vi "Test - Execute Step.vi"(8 "error in (no error)":errorcluster, 11 "Cluster":T1={"Preslip Sequence"=[], "Step No"=0, "Step Value"={"Sr.no"=0, "Log?"=FALSE, "Step"="", "Type"="", "Channel"="", "Value"=0.0, "Para1"=0.0, "Para2"=0.0, "Limit1"=0.0, "Limit2"=0.0, "Comparision Mode"="", "Timeout"=0.0}, "Slip Parameter"=[], "Slip Timer"=0.0, "Postslip Sequence"=[], "Postslip ?"=FALSE, "Step Result"={"Step Name"="", "Value"=0.0, "Success ?"=TRUE, "Stop Seq ?"=TRUE, "Abort"=TRUE, "Sr.No"=0}}) -> (0 "error out":errorcluster, 3 "output cluster":T1={"Preslip Sequence"=[], "Step No"=0, "Step Value"={"Sr.no"=0, "Log?"=FALSE, "Step"="", "Type"="", "Channel"="", "Value"=0.0, "Para1"=0.0, "Para2"=0.0, "Limit1"=0.0, "Limit2"=0.0, "Comparision Mode"="", "Timeout"=0.0}, "Slip Parameter"=[], "Slip Timer"=0.0, "Postslip Sequence"=[], "Postslip ?"=FALSE, "Step Result"={"Step Name"="", "Value"=0.0, "Success ?"=TRUE, "Stop Seq ?"=TRUE, "Abort"=TRUE, "Sr.No"=0}})   [LabVIEW 2017]
uses:
  Test - Message cluster.ctl
  Test - Step config.ctl
  Test - Step Result.ctl
  Controls/RT- Get Set.ctl
  Controls/RT- Queue States.ctl
  DAQ/DAQ -Driver Control.ctl
  SubVIs/SubVI - Global.vi
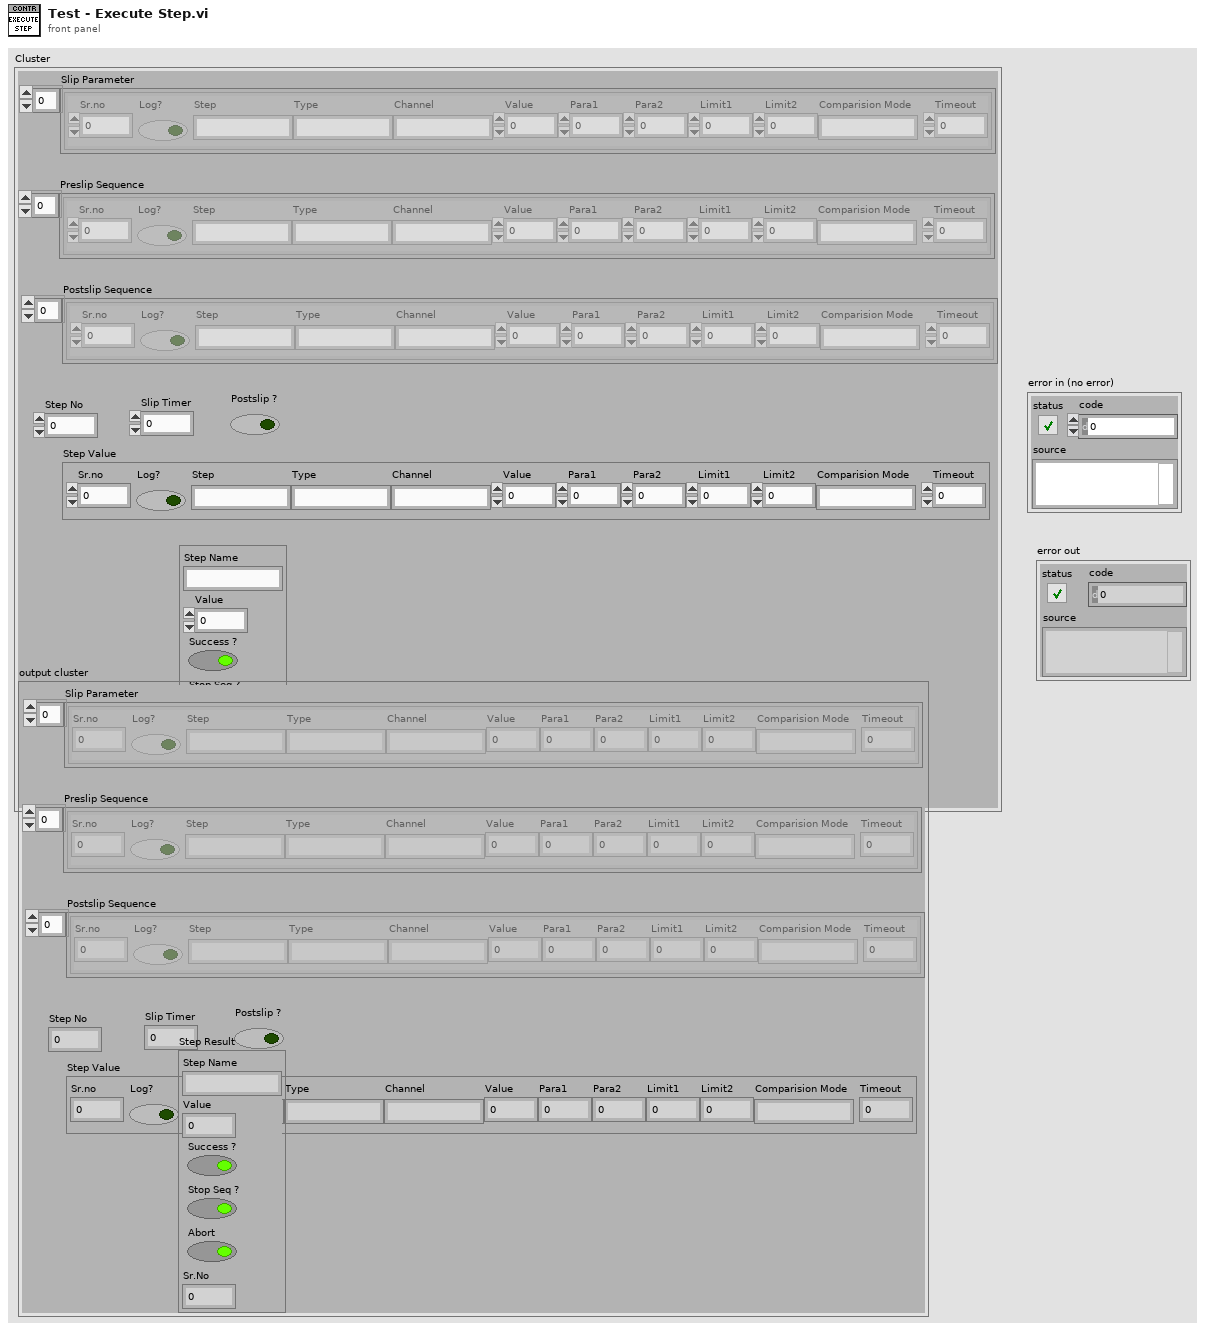
[diagram p1: front panel]
types:
  T1 = typedef "Test - Message cluster.ctl" = cluster{"Preslip Sequence":T2[], "Step No":i32, "Step Value":T2, "Slip Parameter":T2[], "Slip Timer":dbl, "Postslip Sequence":T2[], "Postslip ?":bool, "Step Result":T3}
  T2 = typedef "Test - Step config.ctl" = cluster{"Sr.no":i32, "Log?":bool, "Step":string, "Type":string, "Channel":string, "Value":dbl, "Para1":dbl, "Para2":dbl, "Limit1":dbl, "Limit2":dbl, "Comparision Mode":string, "Timeout":dbl}
  T3 = typedef "Test - Step Result.ctl" = cluster{"Step Name":string, "Value":dbl, "Success ?":bool, "Stop Seq ?":bool, "Abort":bool, "Sr.No":i32}
  T4 = typedef "RT- Get Set.ctl" = enum16{"Reset", "Get", "Set"}
  T5 = typedef "DAQ -Driver Control.ctl" = enum16{"Timeout", "Init", "Config FPGA", "Start Acquisition", "Read Data", "Stop Acquisition", "Flush Queue", "Exit"}
  T6 = typedef "RT- Queue States.ctl" = enum16{"Initialize", "Enqueue", "Enqueue Priority", "Dequeue", "Flush", "Destroy"}
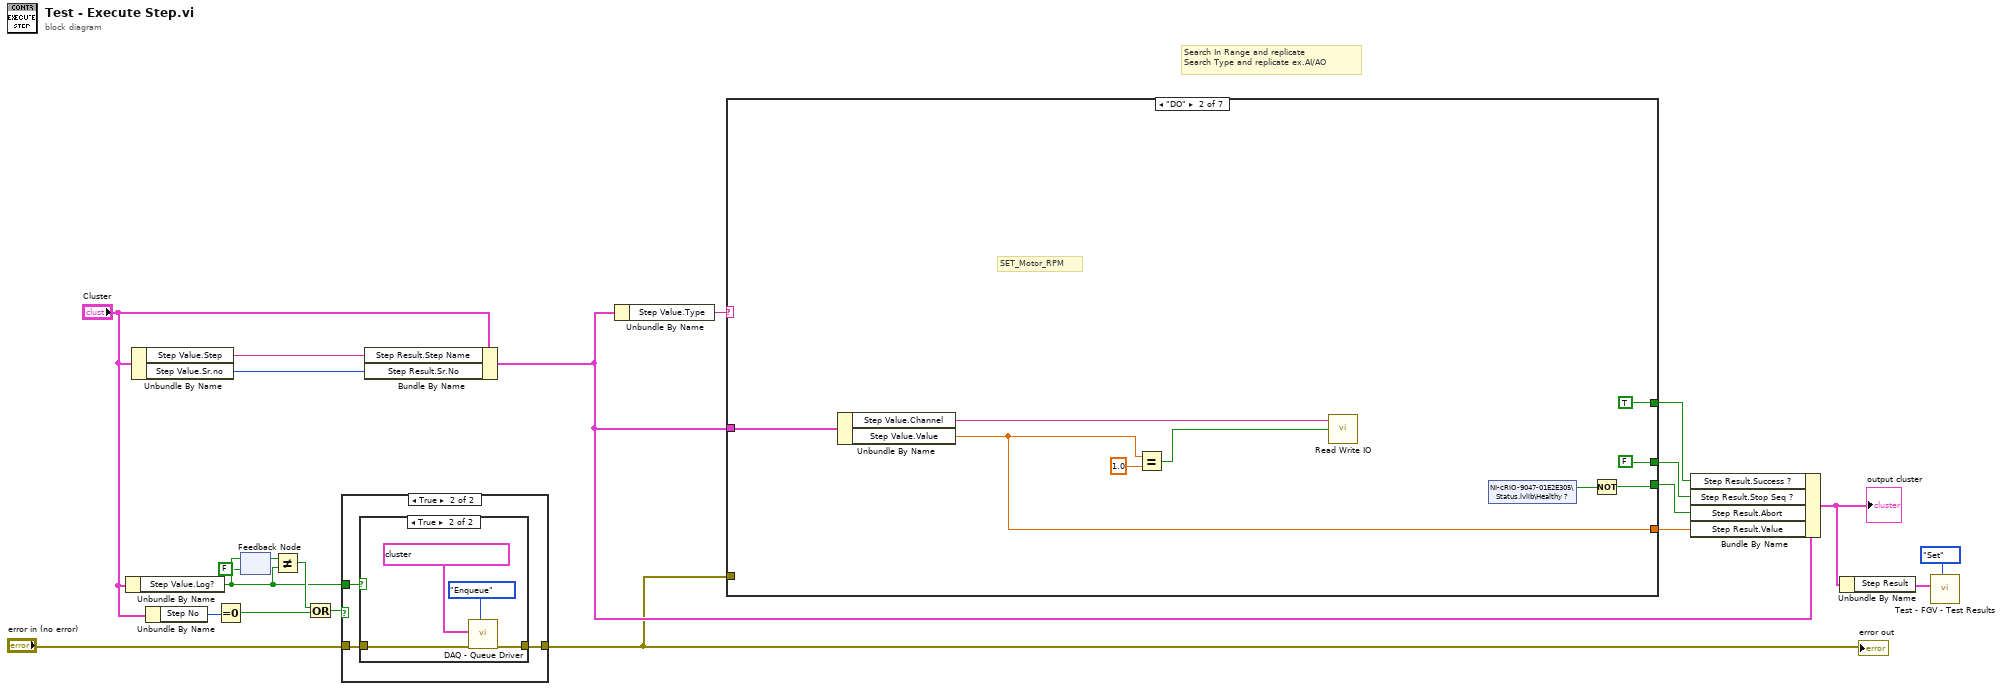
[diagram p0: block diagram]
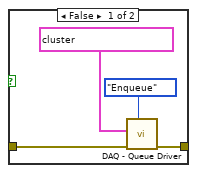
[diagram p3: hidden frame]
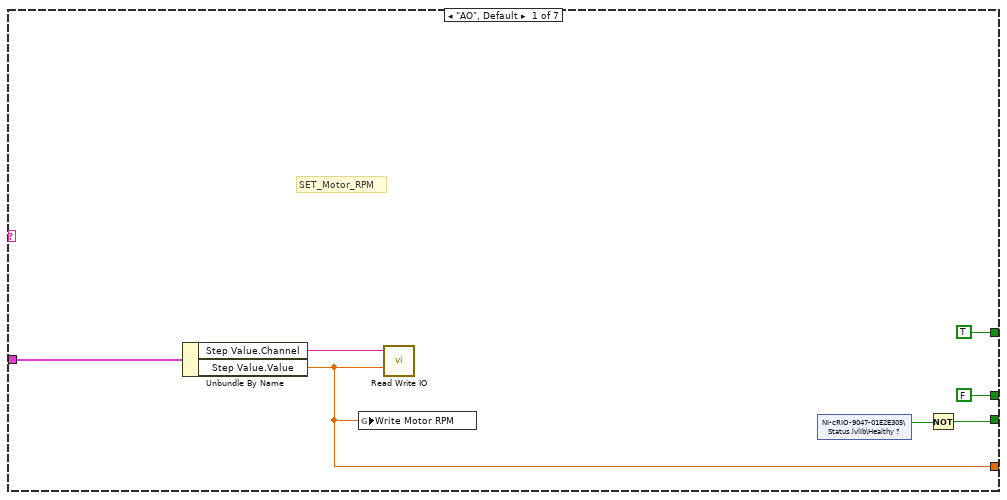
[diagram p4: hidden frame]
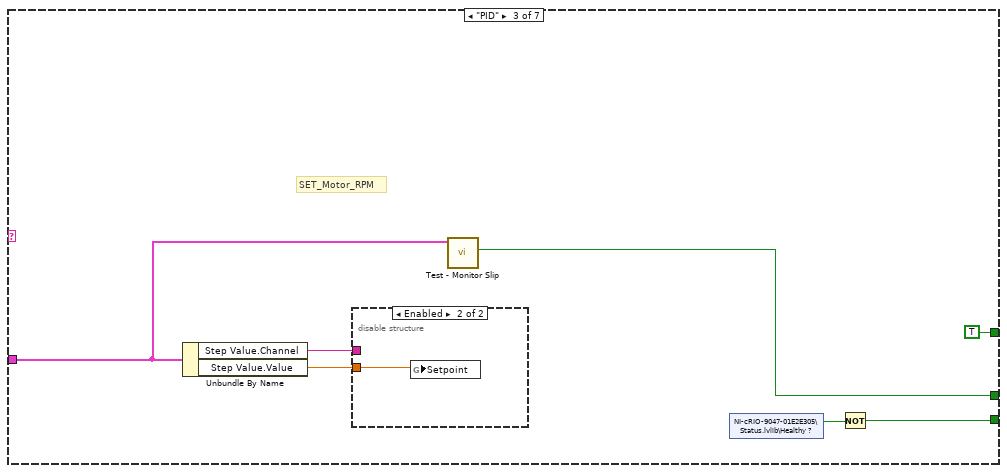
[diagram p5: hidden frame]
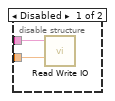
[diagram p6: hidden frame]
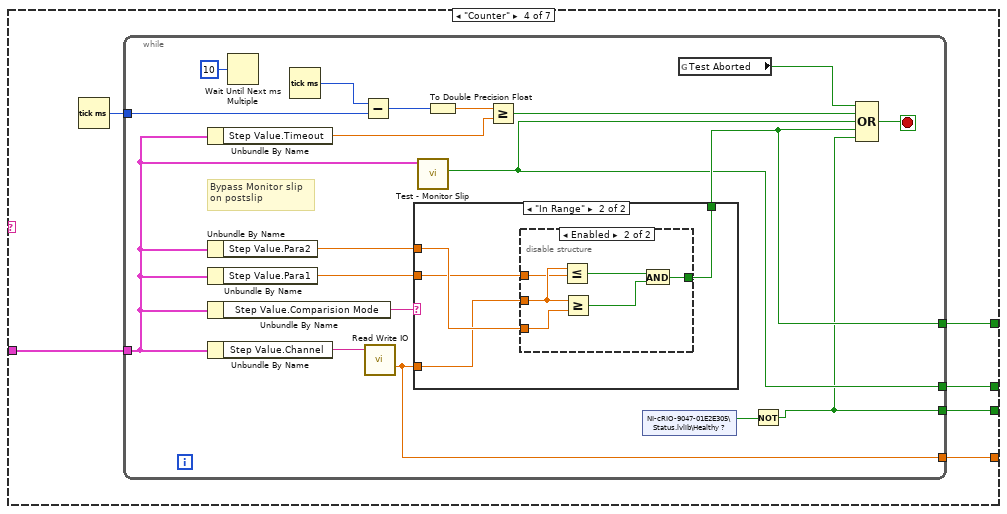
[diagram p7: hidden frame]
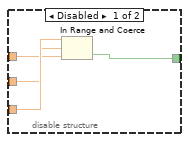
[diagram p9: hidden frame]
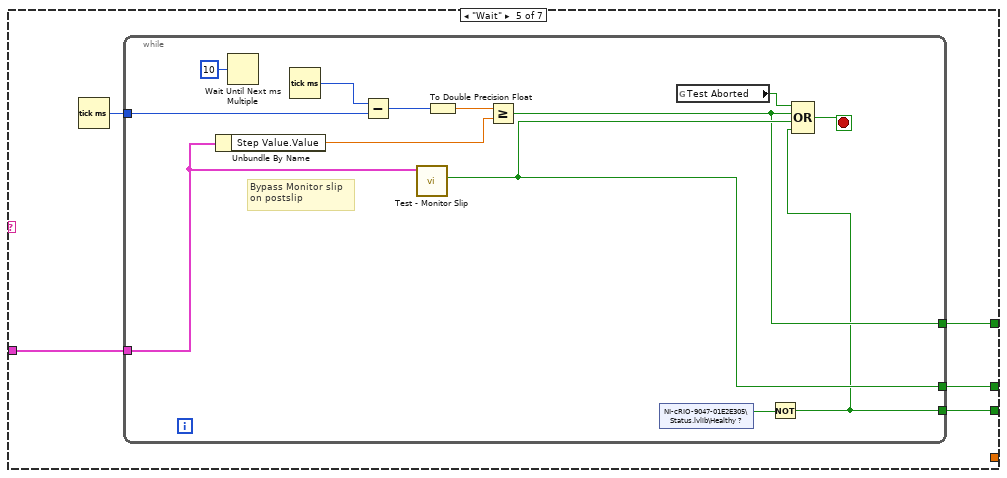
[diagram p10: hidden frame]
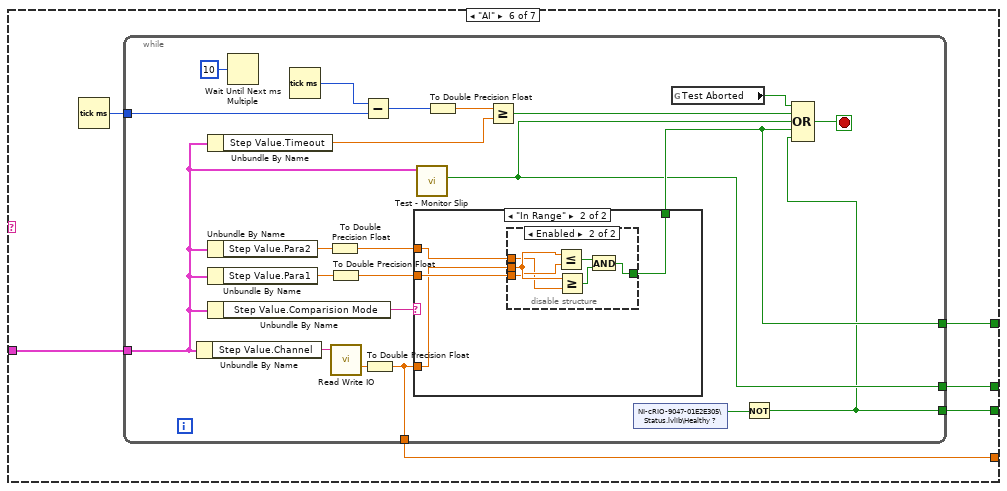
[diagram p11: hidden frame]
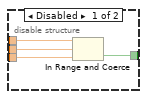
[diagram p13: hidden frame]
diagram:
  # "Search In Range and replicate\nSearch Type and replicate ex.AI/AO"
  n1 = Unbundle By Name("Cluster") -> ("Step Value.Log?"=w4:bool)
  n2 = Unbundle By Name("Cluster") -> ("Step Value.Step"=w13:string, "Step Value.Sr.no"=w1:i32)
  n3 = Unbundle By Name("Cluster") -> ("Step No"=w8:i32)
  n4 = Equal To 0?(x=w8) -> (x = 0?=w7:bool)
  n5 = feedback-in #1(w4) -> ()
  n6 = feedback #1(FALSE ("Log?")) -> (w6:bool)
  n7 = Not Equal?(x=w6, y=w4) -> (x != y?=w5:bool)
  n8 = Or(x=w5, y=w7) -> (x .or. y?=w3:bool)
  n9 = case shown="True" w3 {
    tunnel: "error in (no error)" -> [w22 w25]
    tunnel: [w22 w24] -> w10
    tunnel: w4 -> [_ w23]
    frame False {
    }
    frame True {
      n10 = case shown="True" w23 {
        tunnel: w25 -> [w27 w31]
        tunnel: [w26 w30] -> w24
        frame False {
          n11 = call "DAQ - Queue Driver.vi"("Cases"=RT-_Queue_States."Enqueue", "error in (no error)"=w27, "Element In"=cluster{"Data":variant, "States":T5} {"Data"=variant, "States"=enum."Stop Acquisition"}) -> ("error out"=w26:errorcluster)  [unwired: 6 in, 2 out]
        }
        frame True {
          n12 = call "DAQ - Queue Driver.vi"("Cases"=RT-_Queue_States."Enqueue", "error in (no error)"=w31, "Element In"=cluster{"Data":variant, "States":T5} {"Data"=variant, "States"=enum."Start Acquisition"}) -> ("error out"=w30:errorcluster)  [unwired: 6 in, 2 out]
        }
      }
    }
  }
  "error out" <- w10
  n13 = Bundle By Name(cluster="Cluster", "Step Result.Step Name"=w13, "Step Result.Sr.No"=w1) -> (w12:T1)
  n14 = Unbundle By Name(w12) -> ("Step Value.Type"=w21:string)
  n15 = case shown="\"DO\"" w21 {
    tunnel: w12 -> [w40 w49 w52 w64 w103 w122 _]
    tunnel: [TRUE TRUE TRUE w60 w101 w120 _] -> w19
    tunnel: [w35 w44 w50 w62 w100 w119 _] -> w17
    tunnel: [FALSE FALSE w53 w61 w99 w118 _] -> w18
    tunnel: [w34 w42 _ w63 _ w117 _] -> w20
    tunnel: w10 -> [_ _ _ _ _ _ _]
    frame "AO", Default {
      # "SET_Motor_RPM"
      n16 = Unbundle By Name(w40) -> ("Step Value.Channel"=w39:string, "Step Value.Value"=w34:dbl)
      n17 = global write "SubVI - Global.vi" "Write Motor RPM"(w34) -> ()
      n18 = call "Read Write IO.vi"("Tag Name"=w39, "Value In"=w34) -> ()  [unwired: 11 in, 3 out]
      n19 = shared-variable "NI-cRIO-9047-01E2E305\\Status.lvlib\\Healthy ?"() -> (w36:bool)  [unwired: 1 in, 1 out]
      n20 = Not(x=w36) -> (.not. x?=w35:bool)
    }
    frame "DO" {
      # "SET_Motor_RPM"
      n21 = Unbundle By Name(w49) -> ("Step Value.Channel"=w48:string, "Step Value.Value"=w42:dbl)
      n22 = Equal?(x=w42, y=1.0) -> (x = y?=w41:bool)
      n23 = call "Read Write IO.vi"("Tag Name"=w48, "Value In"=w41) -> ()  [unwired: 11 in, 3 out]
      n24 = shared-variable "NI-cRIO-9047-01E2E305\\Status.lvlib\\Healthy ?"() -> (w45:bool)  [unwired: 1 in, 1 out]
      n25 = Not(x=w45) -> (.not. x?=w44:bool)
    }
    frame "PID" {
      # "SET_Motor_RPM"
      n26 = Unbundle By Name(w52) -> ("Step Value.Channel"=w56:string, "Step Value.Value"=w55:dbl)
      n27 = disable-structure shown="Enabled" {
        disable-tunnel: w56 -> [w58 _]
        disable-tunnel: w55 -> [w57 w59]
        frame Disabled {
          n28 = call "Read Write IO.vi"("Tag Name"=w58, "Value In"=w57) -> ()  [unwired: 11 in, 3 out]
        }
        frame Enabled {
          n29 = global write "SubVI - Global.vi" "Setpoint"(w59) -> ()
        }
      }
      n30 = call "Test - Monitor Slip.vi"("Cluster"=w52) -> ("Slip Occured ?"=w53:bool)  [unwired: 9 in, 1 out]
      n31 = shared-variable "NI-cRIO-9047-01E2E305\\Status.lvlib\\Healthy ?"() -> (w51:bool)  [unwired: 1 in, 1 out]
      n32 = Not(x=w51) -> (.not. x?=w50:bool)
    }
    frame "Counter" {
      n33 = Tick Count (ms)() -> (millisecond timer value=w65:u32)
      n34 = while {
        tunnel: w64 -> [w70]
        tunnel: w65 -> [w79]
        tunnel: [w72] -> w60
        tunnel: [w66] -> w62
        tunnel: [w71] -> w61
        tunnel: [w69] -> w63
        stop <- w74 stop-if-true
        # "Bypass Monitor slip\non postslip"
        n35 = Unbundle By Name(w70) -> ("Step Value.Timeout"=w76:dbl)
        n36 = Unbundle By Name(w70) -> ("Step Value.Para2"=w82:dbl)
        n37 = Unbundle By Name(w70) -> ("Step Value.Para1"=w81:dbl)
        n38 = Unbundle By Name(w70) -> ("Step Value.Comparision Mode"=w83:string)
        n39 = Unbundle By Name(w70) -> ("Step Value.Channel"=w84:string)
        n40 = Wait Until Next ms Multiple(millisecond multiple=u32 10) -> ()  [unwired: 1 out]
        n41 = Tick Count (ms)() -> (millisecond timer value=w78:u32)
        n42 = Subtract(x=w78, y=w79) -> (x-y=w77:u32)
        n43 = call "Read Write IO.vi"("Tag Name"=w84) -> ("Value Out"=w69:dbl)  [unwired: 12 in, 2 out]
        n44 = case shown="\"In Range\"" w83 {
          tunnel: w69 -> [_ w86]
          tunnel: w82 -> [_ w88]
          tunnel: w81 -> [_ w87]
          tunnel: [_ w85] -> w72
          frame "False", Default {
          }
          frame "In Range" {
            n45 = disable-structure shown="Enabled" {
              disable-tunnel: w88 -> [w92 w93]
              disable-tunnel: w87 -> [w91 w94]
              disable-tunnel: w86 -> [w90 w95]
              disable-tunnel: [w89 w96] -> w85
              frame Disabled {
                n46 = In Range and Coerce(upper limit=w92, x=w90, lower limit=w91) -> (In Range?=w89:bool)  [unwired: 1 out]
              }
              frame Enabled {
                n47 = Less Or Equal?(x=w95, y=w94) -> (x <= y?=w97:bool)
                n48 = Greater Or Equal?(x=w95, y=w93) -> (x >= y?=w98:bool)
                n49 = And(x=w97, y=w98) -> (x .and. y?=w96:bool)
              }
            }
          }
        }
        n50 = call "Test - Monitor Slip.vi"("Cluster"=w70) -> ("Slip Occured ?"=w71:bool)  [unwired: 9 in, 1 out]
        n51 = To Double Precision Float(number=w77) -> (double precision float=w73:dbl)
        n52 = Greater Or Equal?(x=w73, y=w76) -> (x >= y?=w75:bool)
        n53 = shared-variable "NI-cRIO-9047-01E2E305\\Status.lvlib\\Healthy ?"() -> (w68:bool)  [unwired: 1 in, 1 out]
        n54 = global read "SubVI - Global.vi" "Test Aborted"() -> (w67:bool)
        n55 = Not(x=w68) -> (.not. x?=w66:bool)
        n56 = Compound Arithmetic op=OR(w67, w75, w71, w72, w66) -> (w74:bool)
      }
    }
    frame "Wait" {
      n57 = Tick Count (ms)() -> (millisecond timer value=w102:u32)
      n58 = while {
        tunnel: w103 -> [w109]
        tunnel: w102 -> [w115]
        tunnel: [w107] -> w101
        tunnel: [w104] -> w100
        tunnel: [w108] -> w99
        stop <- w111 stop-if-true
        # "Bypass Monitor slip\non postslip"
        n59 = Unbundle By Name(w109) -> ("Step Value.Value"=w112:dbl)
        n60 = Wait Until Next ms Multiple(millisecond multiple=u32 10) -> ()  [unwired: 1 out]
        n61 = Tick Count (ms)() -> (millisecond timer value=w114:u32)
        n62 = Subtract(x=w114, y=w115) -> (x-y=w113:u32)
        n63 = call "Test - Monitor Slip.vi"("Cluster"=w109) -> ("Slip Occured ?"=w108:bool)  [unwired: 9 in, 1 out]
        n64 = To Double Precision Float(number=w113) -> (double precision float=w110:dbl)
        n65 = Greater Or Equal?(x=w110, y=w112) -> (x >= y?=w107:bool)
        n66 = shared-variable "NI-cRIO-9047-01E2E305\\Status.lvlib\\Healthy ?"() -> (w106:bool)  [unwired: 1 in, 1 out]
        n67 = global read "SubVI - Global.vi" "Test Aborted"() -> (w105:bool)
        n68 = Not(x=w106) -> (.not. x?=w104:bool)
        n69 = Compound Arithmetic op=OR(w105, w107, w108, w104) -> (w111:bool)
      }
    }
    frame "AI" {
      n70 = Tick Count (ms)() -> (millisecond timer value=w121:u32)
      n71 = while {
        tunnel: w122 -> [w132]
        tunnel: w121 -> [w139]
        tunnel: [w131] -> w120
        tunnel: [w123] -> w119
        tunnel: [w130] -> w118
        tunnel: [w124] -> w117
        stop <- w134 stop-if-true
        n72 = Unbundle By Name(w132) -> ("Step Value.Channel"=w144:string)
        n73 = Unbundle By Name(w132) -> ("Step Value.Timeout"=w136:dbl)
        n74 = Unbundle By Name(w132) -> ("Step Value.Para2"=w142:dbl)
        n75 = Unbundle By Name(w132) -> ("Step Value.Para1"=w141:dbl)
        n76 = Unbundle By Name(w132) -> ("Step Value.Comparision Mode"=w143:string)
        n77 = Wait Until Next ms Multiple(millisecond multiple=u32 10) -> ()  [unwired: 1 out]
        n78 = Tick Count (ms)() -> (millisecond timer value=w138:u32)
        n79 = To Double Precision Float(number=w142) -> (double precision float=w126:dbl)
        n80 = To Double Precision Float(number=w141) -> (double precision float=w125:dbl)
        n81 = call "Read Write IO.vi"("Tag Name"=w144) -> ("Value Out"=w129:dbl)  [unwired: 12 in, 2 out]
        n82 = Subtract(x=w138, y=w139) -> (x-y=w137:u32)
        n83 = To Double Precision Float(number=w129) -> (double precision float=w124:dbl)
        n84 = case shown="\"In Range\"" w143 {
          tunnel: w124 -> [_ w145]
          tunnel: w126 -> [_ w148]
          tunnel: w125 -> [_ w147]
          tunnel: [_ w146] -> w131
          frame "False", Default {
          }
          frame "In Range" {
            n85 = disable-structure shown="Enabled" {
              disable-tunnel: w148 -> [w152 w153]
              disable-tunnel: w147 -> [w151 w154]
              disable-tunnel: [w150 w156] -> w146
              disable-tunnel: w145 -> [w149 w155]
              frame Disabled {
                n86 = In Range and Coerce(upper limit=w152, x=w149, lower limit=w151) -> (In Range?=w150:bool)  [unwired: 1 out]
              }
              frame Enabled {
                n87 = Less Or Equal?(x=w155, y=w154) -> (x <= y?=w157:bool)
                n88 = Greater Or Equal?(x=w155, y=w153) -> (x >= y?=w158:bool)
                n89 = And(x=w157, y=w158) -> (x .and. y?=w156:bool)
              }
            }
          }
        }
        n90 = call "Test - Monitor Slip.vi"("Cluster"=w132) -> ("Slip Occured ?"=w130:bool)  [unwired: 9 in, 1 out]
        n91 = To Double Precision Float(number=w137) -> (double precision float=w133:dbl)
        n92 = Greater Or Equal?(x=w133, y=w136) -> (x >= y?=w135:bool)
        n93 = shared-variable "NI-cRIO-9047-01E2E305\\Status.lvlib\\Healthy ?"() -> (w128:bool)  [unwired: 1 in, 1 out]
        n94 = global read "SubVI - Global.vi" "Test Aborted"() -> (w127:bool)
        n95 = Not(x=w128) -> (.not. x?=w123:bool)
        n96 = Compound Arithmetic op=OR(w127, w135, w130, w131, w123) -> (w134:bool)
      }
    }
    frame "True" {
    }
  }
  n97 = Bundle By Name(cluster=w12, "Step Result.Success ?"=w19, "Step Result.Stop Seq ?"=w18, "Step Result.Abort"=w17, "Step Result.Value"=w20) -> (w15:T1)
  "output cluster" <- w15
  n98 = Unbundle By Name(w15) -> ("Step Result"=w14:T3)
  n99 = call "Test - FGV - Test Results.vi"("Get/Set"=RT-_Get_Set."Set", "Step Result"=w14) -> ()  [unwired: 8 in, 2 out]
